vi "Sprinkler.vi"() -> ()   [LabVIEW 2019]
uses:
  Controls/ControllerStates.ctl
  Controls/InternalData.ctl
  Controls/IndicatorData.ctl
  Controls/TimerStates.ctl
panel:
  in  "Zone Setup Array":cluster{"Zone Selector":string, "Timing":dbl}[](array[cluster])
  out "Controller Status":string
  out "Zone Indicators":T1
  in  "Water Pressure Sensor (%)":u32(slide) scale=0.0..100.0
  in  "Rain Sensor":bool
  in  "Run Selector":bool
  in  "Setup":bool
  in  "Start":bool
  in  "stop":bool
  # "Controls"
  # "Simulation Controls"
  # "Rain"
  # "No Rain"
  # "Continuous"
  # "Single"
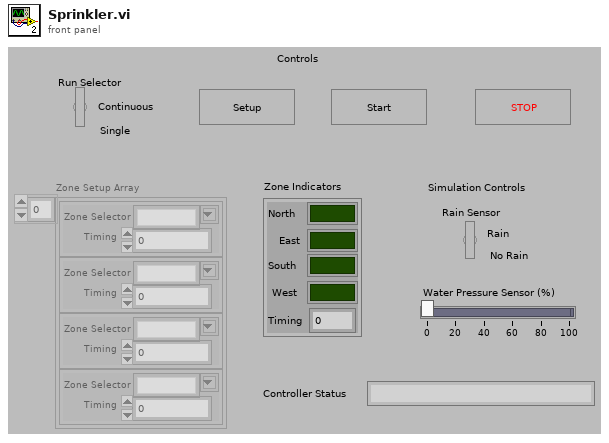
[diagram p1: front panel]
types:
  T1 = cluster{"North":bool, "East":bool, "South":bool, "West":bool, "Timing":u32}
  T2 = typedef "IndicatorData.ctl" = cluster{"Zone Indicators":cluster{"North":bool, "East":bool, "South":bool, "West":bool, "Timing":u32}, "Controller Status":string}
  T3 = typedef "InternalData.ctl" = cluster{"Zone Setup Array":cluster{"Zone Selector":string, "Timing":dbl}[], "CurrentStepID":u32, "ProcessRunning?":bool, "Water Pressure OK?":bool}
  T4 = typedef "ControllerStates.ctl" = enum16{"Initialize", "IDLE", "StartsRun", "ProcessRun", "CheckRun", "StopsRun", "ExitApp"}
  T5 = enum8{"Enabled", "Disabled", "Disabled and Grayed Out"}
  T6 = typedef "TimerStates.ctl" = enum16{"Start", "Read"}
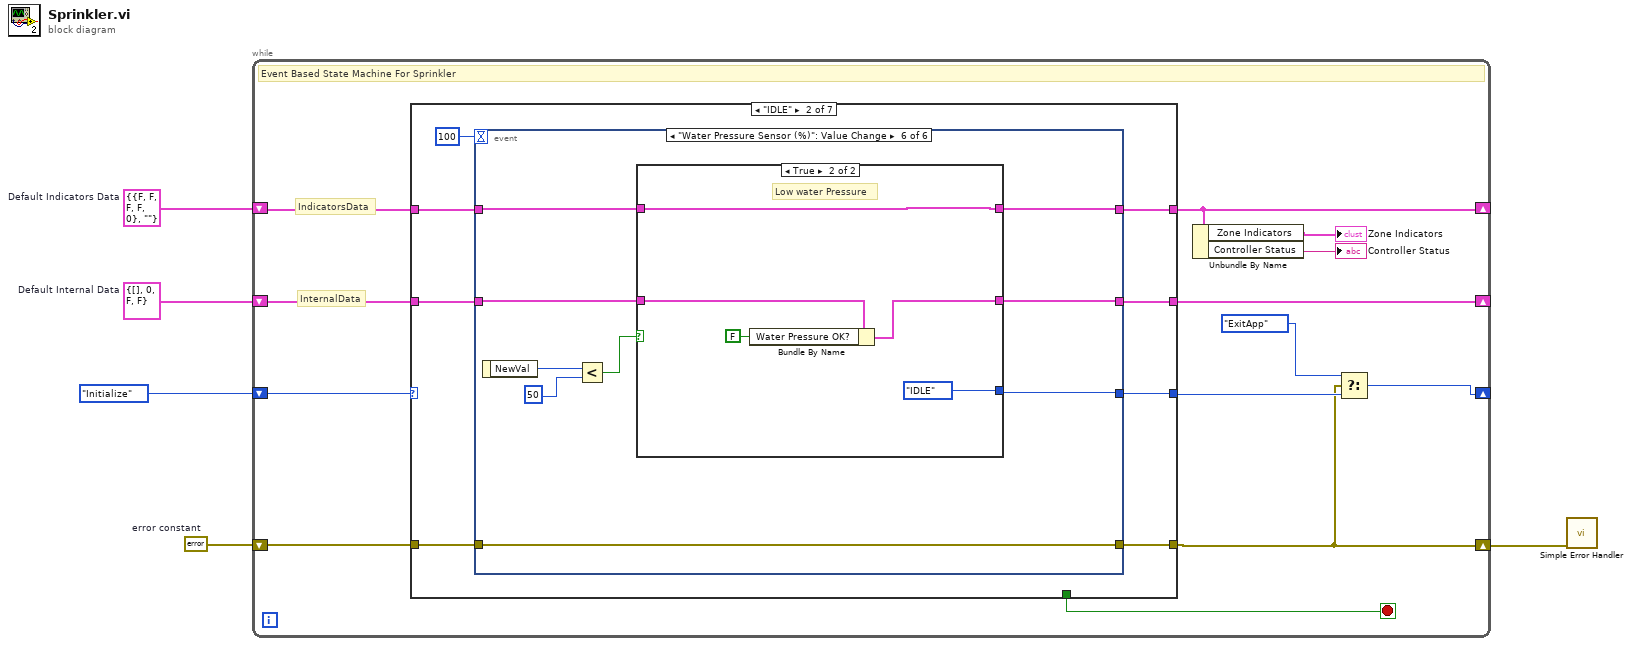
[diagram p0: block diagram]
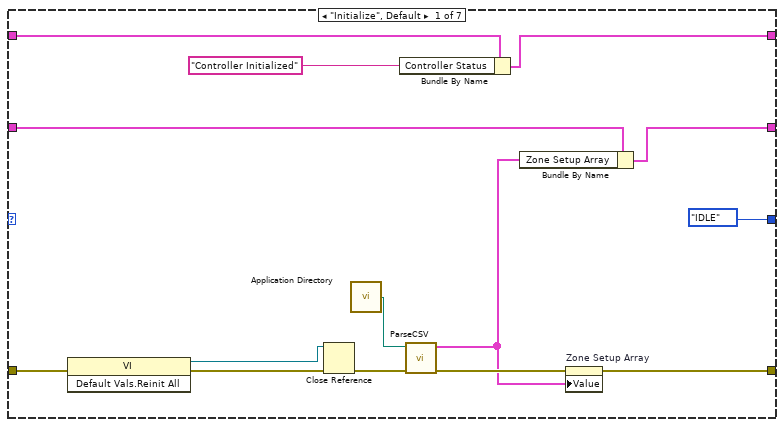
[diagram p2: hidden frame]
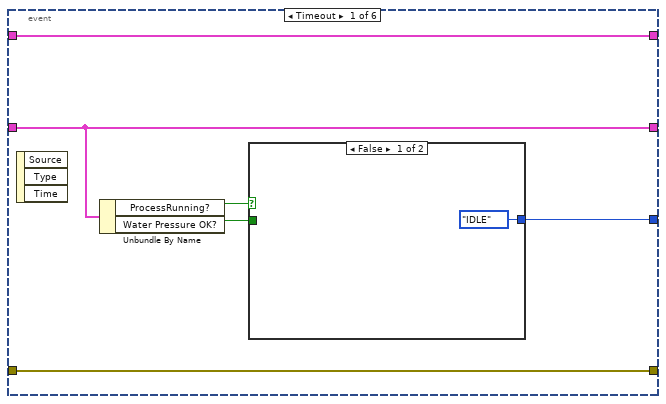
[diagram p3: hidden frame]
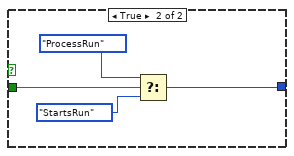
[diagram p4: hidden frame]
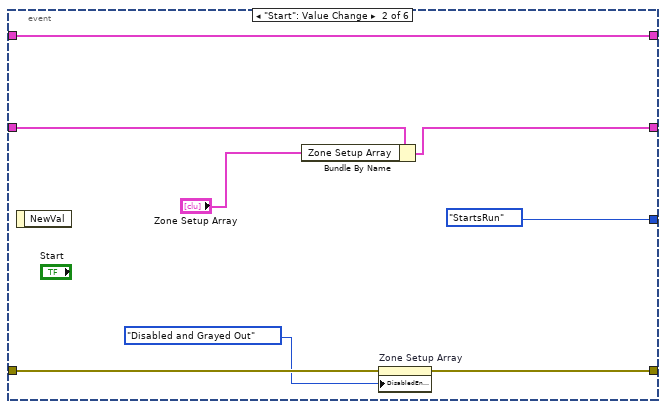
[diagram p5: hidden frame]
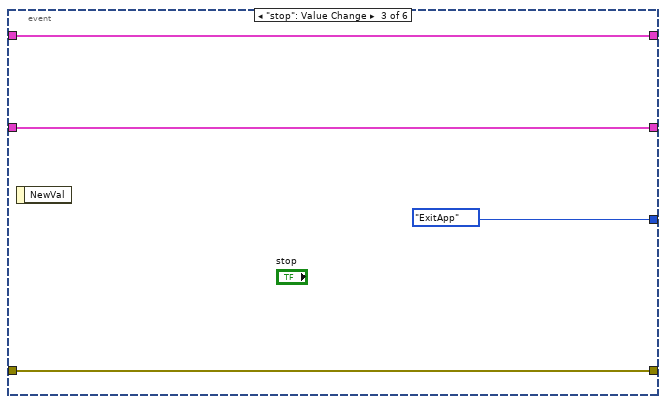
[diagram p6: hidden frame]
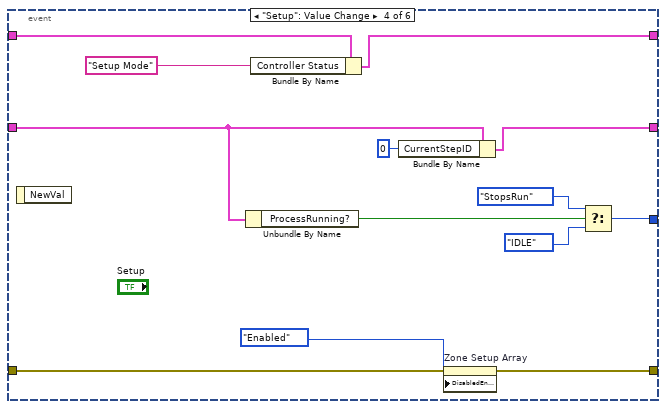
[diagram p7: hidden frame]
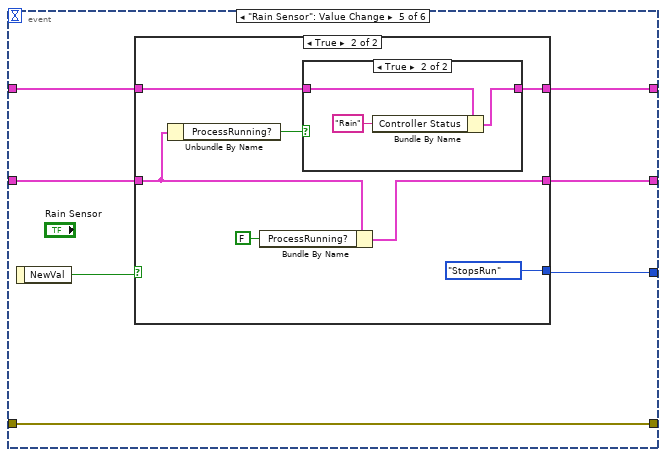
[diagram p8: hidden frame]
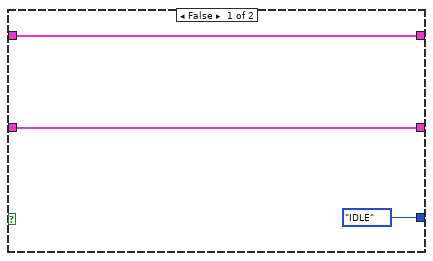
[diagram p9: hidden frame]
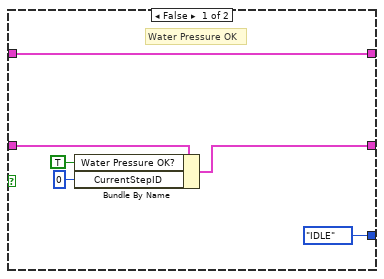
[diagram p11: hidden frame]
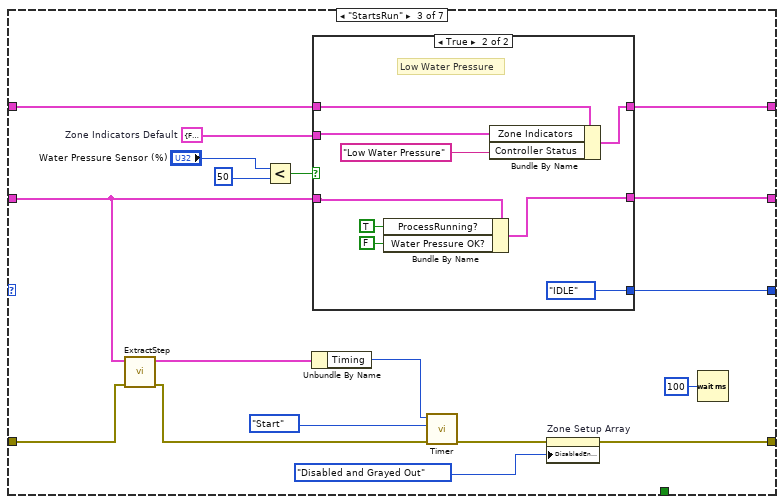
[diagram p12: hidden frame]
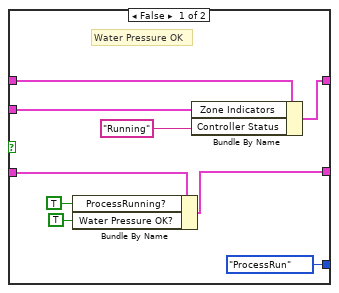
[diagram p13: hidden frame]
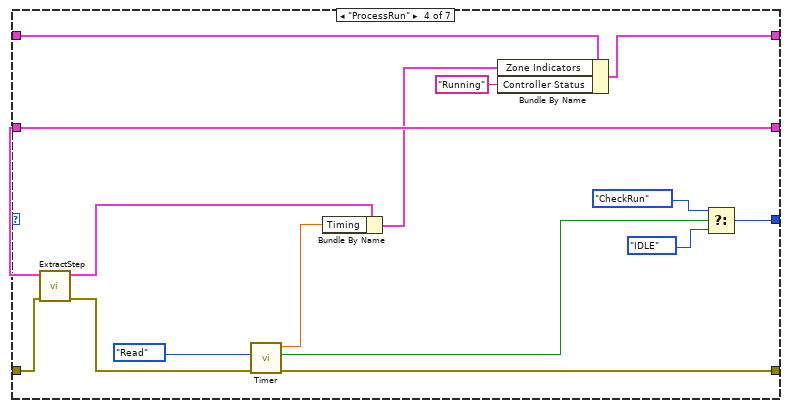
[diagram p14: hidden frame]
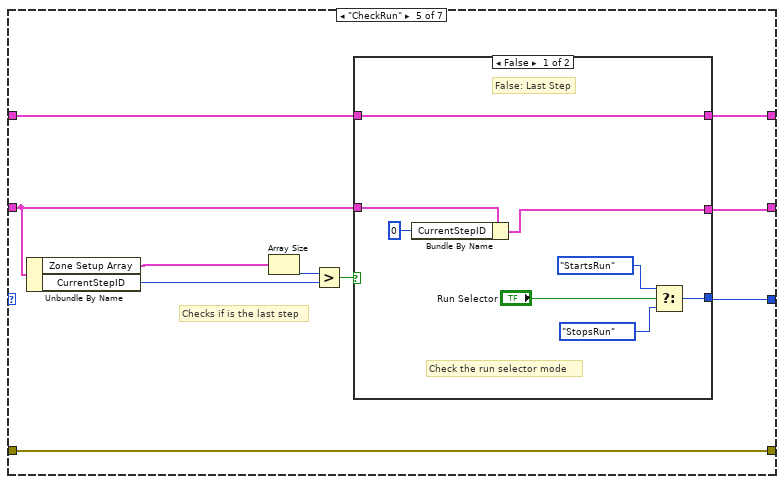
[diagram p15: hidden frame]
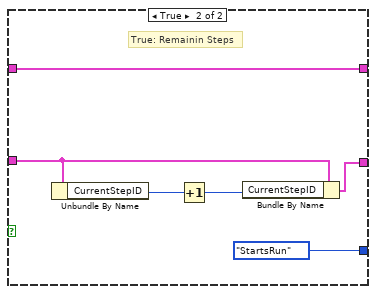
[diagram p16: hidden frame]
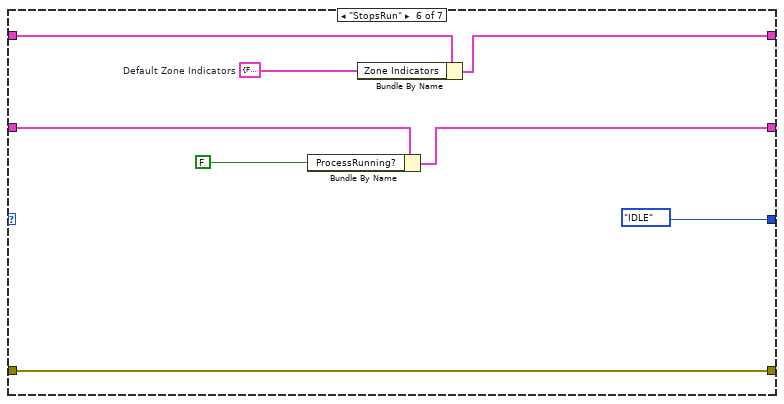
[diagram p17: hidden frame]
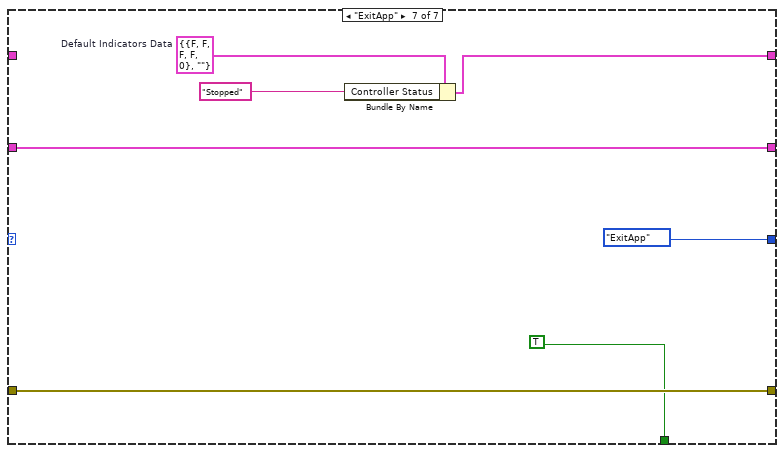
[diagram p18: hidden frame]
diagram:
  w1 = errorcluster {"status"=FALSE, "code"=0, "source"=""}  # error constant
  w4 = T2 {"Zone Indicators"={"North"=FALSE, "East"=FALSE, "South"=FALSE, "West"=FALSE, "Timing"=0}, "Controller Status"=""}  # Default Indicators Data
  w3 = T3 {"Zone Setup Array"=[], "CurrentStepID"=0, "ProcessRunning?"=FALSE, "Water Pressure OK?"=FALSE}  # Default Internal Data
  n1 = while {
    shift-right: [w7] -> w2
    shift-left: w1 -> [w15]
    shift-right: [w14] -> _
    shift-left: w3 -> [w16]
    shift-right: [w13] -> _
    shift-left: w4 -> [w17]
    shift-right: [w8] -> _
    shift-left: ControllerStates."Initialize" -> [w18]
    stop <- w6 stop-if-true
    # "InternalData"
    # "IndicatorsData"
    # "Event Based State Machine For Sprinkler"
    n2 = case shown="\"IDLE\"" w18 {
      tunnel: w17 -> [w21 w37 w123 w157 w170 w195 _]
      tunnel: w16 -> [w23 w35 w120 w159 w172 w197 w206]
      tunnel: w15 -> [w32 w40 w134 w161 w178 w199 w207]
      tunnel: [w25 w39 w129 w162 w178 w199 w207] -> w7
      tunnel: [w19 w36 w122 w156 w169 w193 w202] -> w13
      tunnel: [w22 w34 w119 w159 w171 w196 w206] -> w14
      tunnel: [ControllerStates."IDLE" w38 w121 w166 w174 ControllerStates."IDLE" ControllerStates."ExitApp"] -> w9
      tunnel: [_ _ _ _ _ _ TRUE] -> w6
      frame "Initialize", Default {
        n3 = invoke class="VI" method="Default Vals.Reinit All"(error in=w32) -> (reference out=w30:refnum<vi>, error out=w31:errorcluster)  [unwired: 2 in, 1 out]
        n4 = Close Reference(reference=w30, error in (no error)=w31) -> (error out=w29:errorcluster)
        n5 = call <vilib>:"Application Directory.vi"() -> ("Application Directory"=w28:path)
        n6 = Bundle By Name(cluster=w21, "Controller Status"="Controller Initialized") -> (w19:T2)
        n7 = call "ParseCSV.vi"("error in (no error)"=w29, "Target Path"=w28) -> ("error out"=w26:errorcluster, "Zone Setup Array"=w24:cluster{"Zone Selector":string, "Timing":dbl}[])  [unwired: 8 in]
        n8 = Bundle By Name(cluster=w23, "Zone Setup Array"=w24) -> (w22:T3)
        n9 = property on="Zone Setup Array" class="Arr (strict)"(error in=w26, "Value"=w24) -> (error out=w25:errorcluster)  [unwired: 1 in, 1 out]
      }
      frame "IDLE" {
        n10 = event shown="[5] \"Water Pressure Sensor (%)\": Value Change" {
          selector: _ -> [_ _ _ _ _ _]
          dyn-events: _ -> [_ _ _ _ _ _]
          timeout: 100 -> [_ _ _ _ _ _]
          tunnel: [w46 w55 w63 w75 w83 w106] -> w39
          tunnel: w40 -> [w46 w57 w63 w76 w83 w106]
          tunnel: [w41 ControllerStates."StartsRun" ControllerStates."ExitApp" w70 w82 w101] -> w38
          tunnel: [w45 w59 w60 w67 w81 w100] -> w36
          tunnel: w37 -> [w45 w59 w60 w69 w80 w103]
          tunnel: w35 -> [w44 w54 w61 w66 w77 w98]
          tunnel: [w44 w52 w61 w64 w79 w102] -> w34
          event Timeout {
            n11 = event-data() -> ()  [unwired: 1 in, 3 out]
            n12 = Unbundle By Name(w44) -> ("ProcessRunning?"=w43:bool, "Water Pressure OK?"=w42:bool)
            n13 = case shown="False" w43 {
              tunnel: w42 -> [_ w50]
              tunnel: [ControllerStates."IDLE" ("f") w49] -> w41
              frame False {
              }
              frame True {
                n14 = Select(t=ControllerStates."ProcessRun", s=w50, f=ControllerStates."StartsRun") -> (s? t:f=w49:T4)
              }
            }
          }
          event "Start": Value Change {
            n15 = event-data() -> ()  [unwired: 1 in, 1 out]
            n16 = Bundle By Name(cluster=w54, "Zone Setup Array"="Zone Setup Array") -> (w52:T3)
            n17 = property on="Zone Setup Array" class="Arr (strict)"(error in=w57, "DisabledEnum"=T5."Disabled and Grayed Out" ("Disabled")) -> (error out=w55:errorcluster)  [unwired: 1 in, 1 out]
          }
          event "stop": Value Change {
            n18 = event-data() -> ()  [unwired: 1 in, 1 out]
          }
          event "Setup": Value Change {
            n19 = event-data() -> ()  [unwired: 1 in, 1 out]
            n20 = Unbundle By Name(w66) -> ("ProcessRunning?"=w71:bool)
            n21 = Bundle By Name(cluster=w69, "Controller Status"="Setup Mode") -> (w67:T2)
            n22 = Bundle By Name(cluster=w66, "CurrentStepID"=u32 0) -> (w64:T3)
            n23 = property on="Zone Setup Array" class="Arr (strict)"(error in=w76, "DisabledEnum"=T5."Enabled" ("Disabled")) -> (error out=w75:errorcluster)  [unwired: 1 in, 1 out]
            n24 = Select(t=ControllerStates."StopsRun", s=w71, f=ControllerStates."IDLE") -> (s? t:f=w70:T4)
          }
          event "Rain Sensor": Value Change {
            n25 = event-data() -> ("NewVal"=w78:bool)  [unwired: 1 in]
            n26 = case shown="True" w78 {
              tunnel: [ControllerStates."IDLE" ControllerStates."StopsRun"] -> w82
              tunnel: [w84 w91] -> w81
              tunnel: w80 -> [w84 w92]
              tunnel: [w85 w87] -> w79
              tunnel: w77 -> [w85 w89]
              frame False {
              }
              frame True {
                n27 = Unbundle By Name(w89) -> ("ProcessRunning?"=w90:bool)
                n28 = Bundle By Name(cluster=w89, "ProcessRunning?"=FALSE) -> (w87:T3)
                n29 = case shown="True" w90 {
                  tunnel: [w94 w96] -> w91
                  tunnel: w92 -> [w94 w95]
                  frame False {
                  }
                  frame True {
                    n30 = Bundle By Name(cluster=w95, "Controller Status"="Rain") -> (w96:T2)
                  }
                }
              }
            }
          }
          event "Water Pressure Sensor (%)": Value Change {
            n31 = event-data() -> ("NewVal"=w105:u32)  [unwired: 1 in]
            n32 = Less?(x=w105, y=u32 50) -> (x < y?=w99:bool)
            n33 = case shown="True" w99 {
              tunnel: [ControllerStates."IDLE" ControllerStates."IDLE"] -> w101
              tunnel: [w112 w113] -> w100
              tunnel: w103 -> [w112 w113]
              tunnel: [w108 w114] -> w102
              tunnel: w98 -> [w110 w116]
              frame False {
                # "Water Pressure OK"
                n34 = Bundle By Name(cluster=w110, "Water Pressure OK?"=TRUE, "CurrentStepID"=u32 0) -> (w108:T3)
              }
              frame True {
                # "Low water Pressure"
                n35 = Bundle By Name(cluster=w116, "Water Pressure OK?"=FALSE) -> (w114:T3)
              }
            }
          }
        }
      }
      frame "StartsRun" {
        w124 = T1 {"North"=FALSE, "East"=FALSE, "South"=FALSE, "West"=FALSE, "Timing"=0}  # Zone Indicators Default
        n36 = call "ExtractStep.vi"("error in (no error)"=w134, "Internal Data"=w120) -> ("error out"=w133:errorcluster, "Zone Indicators Default"=w132:T1)  [unwired: 8 in]
        n37 = Less?(x="Water Pressure Sensor (%)", y=u32 50) -> (x < y?=w125:bool)
        n38 = Unbundle By Name(w132) -> ("Timing"=w131:u32)
        n39 = case shown="True" w125 {
          tunnel: w124 -> [w141 w152]
          tunnel: [w142 w151] -> w122
          tunnel: w123 -> [w143 w150]
          tunnel: [ControllerStates."ProcessRun" ControllerStates."IDLE"] -> w121
          tunnel: w120 -> [w140 w148]
          tunnel: [w138 w146] -> w119
          frame False {
            # "Water Pressure OK"
            n40 = Bundle By Name(cluster=w140, "ProcessRunning?"=TRUE, "Water Pressure OK?"=TRUE) -> (w138:T3)
            n41 = Bundle By Name(cluster=w143, "Zone Indicators"=w141, "Controller Status"="Running") -> (w142:T2)
          }
          frame True {
            # "Low Water Pressure"
            n42 = Bundle By Name(cluster=w148, "ProcessRunning?"=TRUE ("Water Pressure OK?"), "Water Pressure OK?"=FALSE) -> (w146:T3)
            n43 = Bundle By Name(cluster=w150, "Zone Indicators"=w152, "Controller Status"="Low Water Pressure") -> (w151:T2)
          }
        }
        n44 = call "Timer.vi"("error in (no error)"=w133, "Timer Command"=TimerStates."Start", "Time Target (s)"=w131) -> ("error out"=w130:errorcluster)  [unwired: 6 in, 2 out]
        n45 = property on="Zone Setup Array" class="Arr (strict)"(error in=w130, "DisabledEnum"=T5."Disabled and Grayed Out" ("Disabled")) -> (error out=w129:errorcluster)  [unwired: 1 in, 1 out]
        n46 = Wait (ms)(milliseconds to wait=u32 100) -> ()  [unwired: 1 out]
      }
      frame "ProcessRun" {
        n47 = call "ExtractStep.vi"("error in (no error)"=w161, "Internal Data"=w159) -> ("error out"=w160:errorcluster, "Zone Indicators Default"=w158:T1)  [unwired: 8 in]
        n48 = call "Timer.vi"("error in (no error)"=w160, "Timer Command"=TimerStates."Read") -> ("error out"=w162:errorcluster, "Time has Elapsed"=w164:bool, "Elapsed Time (s)"=w168:dbl)  [unwired: 7 in]
        n49 = Bundle By Name(cluster=w158, "Timing"=w168) -> (w155:T1)
        n50 = Bundle By Name(cluster=w157, "Zone Indicators"=w155, "Controller Status"="Running") -> (w156:T2)
        n51 = Select(t=ControllerStates."CheckRun", s=w164, f=ControllerStates."IDLE") -> (s? t:f=w166:T4)
      }
      frame "CheckRun" {
        # "Checks if is the last step"
        n52 = Unbundle By Name(w172) -> ("Zone Setup Array"=w177:cluster{"Zone Selector":string, "Timing":dbl}[], "CurrentStepID"=w175:u32)
        n53 = Array Size(array=w177) -> (size(s)=w176:i32)
        n54 = Greater?(x=w176, y=w175) -> (0:w173:bool)
        n55 = case shown="False" w173 {
          tunnel: [w186 ControllerStates."StartsRun"] -> w174
          tunnel: [w180 w191] -> w171
          tunnel: w172 -> [w182 w190]
          tunnel: w170 -> [w179 w187]
          tunnel: [w179 w187] -> w169
          frame False {
            # "Check the run selector mode"
            # "False: Last Step"
            n56 = Bundle By Name(cluster=w182, "CurrentStepID"=u32 0 ("CurrentZoneID")) -> (w180:T3)
            n57 = Select(t=ControllerStates."StartsRun", s="Run Selector", f=ControllerStates."StopsRun") -> (s? t:f=w186:T4)
          }
          frame True {
            # "True: Remainin Steps"
            n58 = Unbundle By Name(w190) -> ("CurrentStepID"=w189:u32)
            n59 = Increment(x=w189) -> (x+1=w188:u32)
            n60 = Bundle By Name(cluster=w190, "CurrentStepID"=w188) -> (w191:T3)
          }
        }
      }
      frame "StopsRun" {
        w194 = T1 {"North"=FALSE, "East"=FALSE, "South"=FALSE, "West"=FALSE, "Timing"=0}  # Default Zone Indicators
        n61 = Bundle By Name(cluster=w197, "ProcessRunning?"=FALSE) -> (w196:T3)
        n62 = Bundle By Name(cluster=w195, "Zone Indicators"=w194) -> (w193:T2)
      }
      frame "ExitApp" {
        w203 = T2 {"Zone Indicators"={"North"=FALSE, "East"=FALSE, "South"=FALSE, "West"=FALSE, "Timing"=0}, "Controller Status"=""}  # Default Indicators Data
        n63 = Bundle By Name(cluster=w203, "Controller Status"="Stopped") -> (w202:T2)
      }
    }
    n64 = Unbundle By Name(w13) -> ("Zone Indicators"=→"Zone Indicators":T1, "Controller Status"=→"Controller Status":string)
    n65 = Select(t=ControllerStates."ExitApp", s=w7, f=w9) -> (s? t:f=w8:T4)
  }
  n66 = call <vilib>:"Simple Error Handler.vi"("error in (no error)"=w2) -> ()  [unwired: 4 in, 5 out]
